vi "StrShuffle.vi"(1 "String in":string) -> (0 "String shuffled":string)   [LabVIEW 2010]
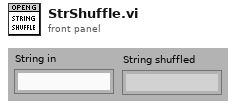
[diagram p1: front panel]
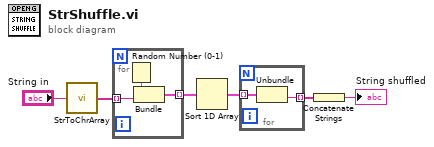
[diagram p0: block diagram]
diagram:
  n1 = call "StrToChrArray.vi"("String in"="String in") -> ("Array char"=w5:string[])
  n2 = for {
    tunnel: w5 -> [w9] mode=indexing
    tunnel: [w7] -> w4 mode=indexing
    n3 = Random Number (0-1)() -> (number: 0 to 1=w8:dbl)
    n4 = Bundle("number: 0 to 1"=w8, "String"=w9) -> (w7:cluster{"number: 0 to 1":dbl, "String":string})  [unwired: 1 in]
  }
  n5 = Sort 1D Array(array=w4) -> (sorted array=w3:cluster{"number: 0 to 1":dbl, "String":string}[])
  n6 = for {
    tunnel: w3 -> [w11] mode=indexing
    tunnel: [w10] -> w2 mode=indexing
    n7 = Unbundle(w11) -> ("String"=w10:string)  [unwired: 1 out]
  }
  n8 = Concatenate Strings(w2) -> (→"String shuffled":string)
